vi "Load_from_Project.vi"(8 "error in (no error)":errorcluster, 9 "index":i32, 10 "buildObject":T3, 11 "AB_Source_Exported_Assembly_VI in":refnum<class "AB_Source_Exported_Assembly_VI.lvclass">) -> (0 "error out":errorcluster, 2 "linker info":T2, 3 "AB_Source_Exported_Assembly_VI out":refnum<class "AB_Source_Exported_Assembly_VI.lvclass">)   [LabVIEW 2020, in "AB_Source_Exported_Assembly_VI.lvclass"]
uses:
  <vilib>/AppBuilder/AB_Classes/Source/ExportedAssemblyVI/AB_Source_Exported_Assembly_VI.lvclass
  <resource>/Framework/Providers/API/ItemRef.ctl
  <vilib>/Utility/lvfile.llb/LVFileType.ctl
  <vilib>/AppBuilder/RW_Project/AB_RW_Project_PropBag_Action.ctl
  <vilib>/AppBuilder/AB_Classes/Source/ExportedAssemblyVI/AB_Source_Exported_Assembly_VI.lvclass/AB_Source_Exported_Assembly_VI.ctl
  <vilib>/AppBuilder/AB_Classes/Source/VI/AB_Source_VI.lvclass
  <vilib>/Utility/lvfile.llb/NI_FileType.lvlib
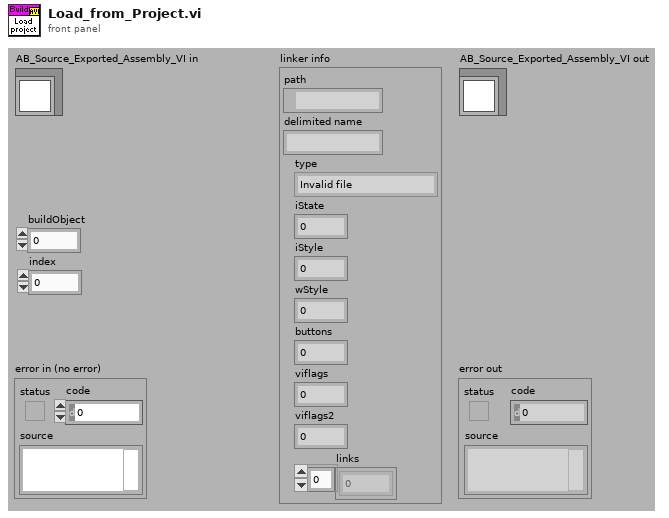
[diagram p1: front panel]
types:
  T1 = typedef "NI_FileType.lvlib/LVFileType.ctl" = enum32{"Invalid file", "Unknown type", "Instrument", "Control", "Polymorphic VI", "Project", "Library", "LVClass", "XControl", "XNode", "Shared library", ".NET assembly", "ActiveX interface", "CIN", "Run-time menu", "Palette menu", "Help file", "LLB", "XNode Edit Dependency", "Class Private Data Control", "Statechart", "MathScript .m file", "Ladder Diagram", "LVLibp", "XNode Build Dependency"}
  T2 = cluster{"path":path, "delimited name":string, "type":T1, "iState":u32, "iStyle":u16, "wStyle":u16, "buttons":u16, "viflags":u32, "viflags2":u32, "links":u32[]}
  T3 = typedef "ItemRef.ctl" = u64
  T4 = typedef "AB_RW_Project_PropBag_Action.ctl" = enum16{"read", "write", "clear", "readPrevious", "writePrevious", "clearPrevious"}
  T5 = typedef "AB_RW_Project_Source_ExportedAssemblyVI_Data.ctl" = cluster{"ExportAssemblyVIinfo":T6}
  T6 = typedef "AB_InteropAssembly_DistVI_Proto_Info.ctl" = cluster{"Library Name":string, "VI Name":string, "Method Name":string, "LV Class":path, "Param Names":string[], "Data Types":string[], "Dirs":T7[], "InputIdx":i32[], "OutputIdx":i32[], "ConNum":i8[], "IsCustomDocumentation":bool, "Custom Documentation":string, "IsProtected":bool, "IsSanitized":bool}
  T7 = typedef "IOStatus.ctl" = enum16{"Input", "Output", "Input/Output", "InputDeleted", "OutputDeleted", "IODeleted", "ErrorClusterIn", "ErrorClusterOut"}
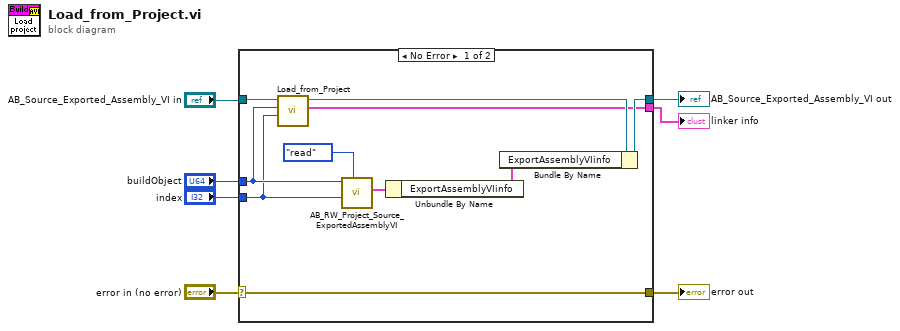
[diagram p0: block diagram]
diagram:
  n1 = case shown="No Error" "error in (no error)" {
    selector: "error in (no error)" -> [w16 w18]
    tunnel: "AB_Source_Exported_Assembly_VI in" -> [w17 w19]
    tunnel: [w14 w19] -> w5
    tunnel: [w16 w18] -> w4
    tunnel: "buildObject" -> [w12 _]
    tunnel: "index" -> [w11 _]
    tunnel: [w8 _] -> w1
    frame No Error {
      n2 = call-parent "Load_from_Project.vi"("index"=w11, "buildObject"=w12, "AB_Source_VI in"=w17) -> ("linker info"=w8:T2, "AB_Source_VI out"=w15:refnum<class "AB_Source_Exported_Assembly_VI.lvclass">)  [unwired: 1 in, 6 out]
      n3 = call <vilib>:"AB_RW_Project_Source_ExportedAssemblyVI.vi"("action"=AB_RW_Project_PropBag_Action."read", "index in"=w11, "buildObject"=w12) -> ("dataSource out"=w9:T5)  [unwired: 2 in, 6 out]
      n4 = Unbundle By Name(w9) -> ("ExportAssemblyVIinfo"=w13:T6)
      n5 = Bundle By Name(cluster=w15, "ExportAssemblyVIinfo"=w13) -> (w14:refnum<class "AB_Source_Exported_Assembly_VI.lvclass">)
    }
    frame Error {
    }
  }
  "error out" <- w4
  "AB_Source_Exported_Assembly_VI out" <- w5
  "linker info" <- w1
